vi "Send Configure Number of Averages [AA].vi"(7 "Message Priority (Normal)":T1=enum."Normal", 8 "error in (no error)":errorcluster, 10 "number of averages (8)":i32=8, 11 "Message Enqueuer":refnum<class "Message Enqueuer.lvclass">) -> (0 "error out":errorcluster, 3 "Message Enqueuer out":refnum<class "Message Enqueuer.lvclass">)   [LabVIEW 2016, in "CS++Scope.lvlib" / "Configure Number of Averages [AA] Msg.lvclass"]
doc: "Sends the <B>CS++Scope.lvlib:Configure Number of Averages [AA] Msg.lvclass</B> message.\n\n<B>CS++Scope.lvlib:CS++Scope.lvclass:Configure Number of Averages [AA].vi</B> Description:\n\nWhen you set the acquisition type to IVISCOPE_VAL_AVERAGE, the oscilloscope acquires multiple waveforms. After each waveform acquisition, the oscilloscope keeps the average value of all acquisitions for each element in the waveform record. This VI configures the number of waveforms that the oscilloscope acquires and averages. After the oscilloscope acquires as many waveforms as you specify, it returns to the idle state."
uses:
  Configure Number of Averages [AA] Msg.lvclass
  <vilib>/ActorFramework/Message Enqueuer/Message Enqueuer.lvclass
  <vilib>/ActorFramework/Message Enqueuer/Message Priority.ctl
  C:/Program Files (x86)/National Instruments/LabVIEW 2016/vi.lib/ActorFramework/Message/Message.lvclass
  Configure Number of Averages [AA] Msg.lvclass/Configure Number of Averages [AA] Msg.ctl
  <vilib>/ActorFramework/Message Enqueuer/Message Enqueuer.lvclass/Message Enqueuer.ctl
  <vilib>/ActorFramework/Message Priority Queue/Priority Enqueue.vi
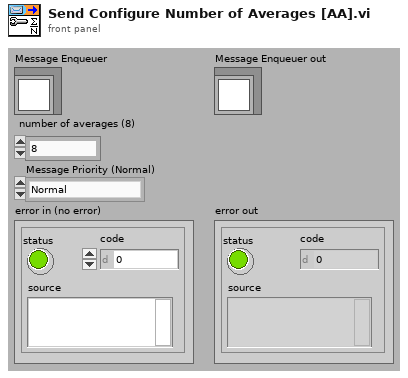
[diagram p1: front panel]
types:
  T1 = typedef "Actor Framework.lvlib/Message Enqueuer.lvclass/Message Priority.ctl" = enum16{"Low", "Normal", "High"}
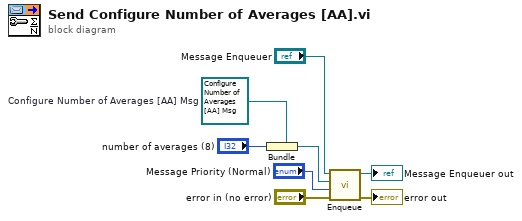
[diagram p0: block diagram]
diagram:
  w2 = refnum<class "Configure Number of Averages [AA] Msg.lvclass"> refnum  # Configure Number of Averages [AA] Msg
  n1 = Bundle(cluster=w2, "number of averages (8)") -> (w5:refnum<class "Configure Number of Averages [AA] Msg.lvclass">)
  n2 = call <vilib>:"Enqueue.vi"("error in (no error)"="error in (no error)", "Message Priority (Normal)"="Message Priority (Normal)", "Message"=w5, "Message Enqueuer in"="Message Enqueuer") -> ("error out"=→"error out":errorcluster, "Message Enqueuer out"=→"Message Enqueuer out":refnum<class "Message Enqueuer.lvclass">)  [unwired: 6 in]
